vi "Get_PV-I.vi"(0 "CA Lab data":T2, 11 "Error in (no error)":errorcluster) -> (4 "PV Name (dup)":string, 6 "1rst Value (string)":string, 8 "1rst Value (number)":dbl, 10 "Value Array (number)":dbl[](array[numeric]), 13 "Status":bool, 14 "PV Info":T1[](array[typedef]), 15 "Error out":errorcluster)   [LabVIEW 2018]
doc: "This is a VI for reading values of EPICS variables.\n\nINPUT:\n <b>CA Lab data</b>\n Cluster with preinitialized data\n <b>Error in (no error)</b>\n\nOUTPUT:\n <b>PV Name (dup)</b>\n name array of EPICS variables\n <b>1st Value(string)</b>\n value of variable as String\n shows first item of value array\n <b>1st Value(number)</b>\n value of variable as Double\n shows first item of value array\n <b>Value Array(number)</b>\n all values of variable in Double array\n <b>Error out</b>\n <b>PV Info</b>\n cluster array of full answer\n value array(number)\n PV name\n elements\n size of value array\n value array(string)\n all values of variable in string array\n value array(number)\n elements\n size of value array\n status(string)\n status of EPICS PV as String\n status(number)\n status of EPICS PV as Long\n severity(string)\n severity of EPICS PV as String\n severity(number)\n severity of EPICS PV as Long\n time stamp(string)\n stamp of EPICS PV time as String\n time stamp(number)\n stamp of EPICS PV as Long\n field names\n field values\n string array of requsted EPICS field values\n error IO\n <b>Status</b>\n FALSE: request successful\n TRUE: warnings or errors"
uses:
  <userlib>/caLab/PV Info.ctl
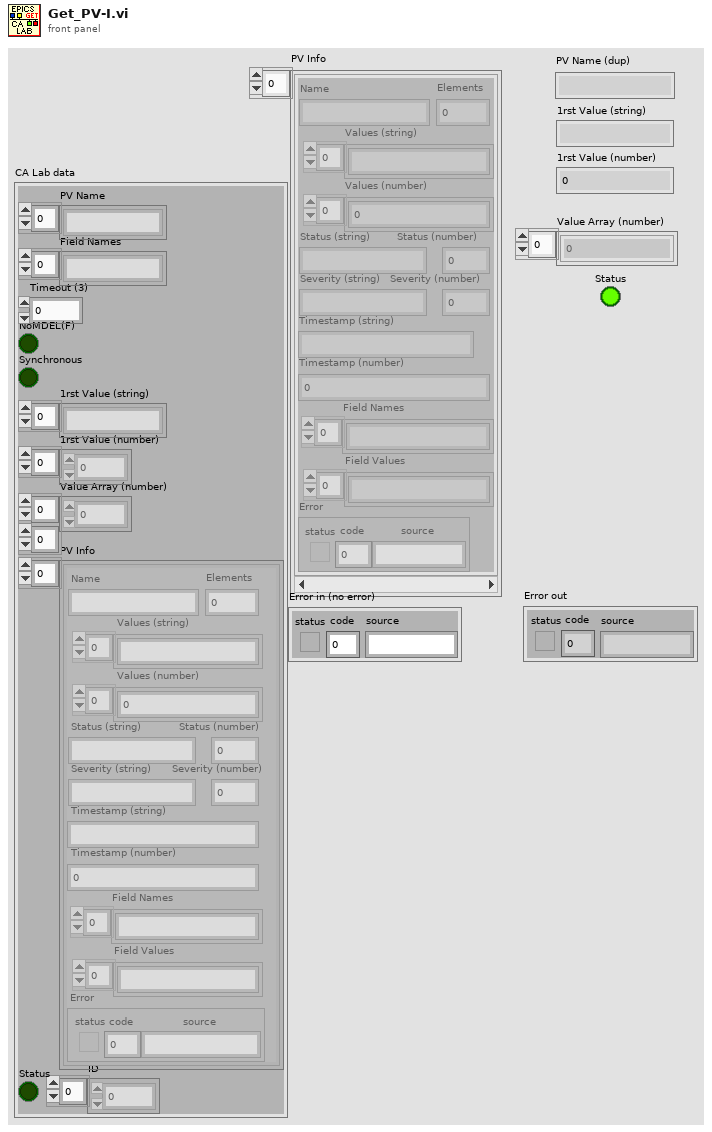
[diagram p1: front panel]
types:
  T1 = typedef "PV Info.ctl" = cluster{"Name":string, "Elements":i32, "Values (string)":string[], "Values (number)":dbl[], "Status (string)":string, "Status (number)":i16, "Severity (string)":string, "Severity (number)":i16, "Timestamp (string)":string, "Timestamp (number)":i32, "Field Names":string[], "Field Values":string[], "Error":errorcluster}
  T2 = cluster{"PV Name":string[], "Field Names":string[], "Timeout (3)":dbl, "NoMDEL(F)":bool, "Synchronous":bool, "1rst Value (string)":string[], "1rst Value (number)":dbl[], "Value Array (number)":dbl[][], "PV Info":T1[], "Status":bool, "ID":u64[]}
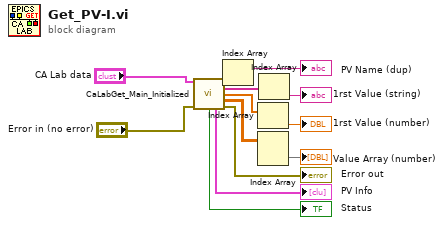
[diagram p0: block diagram]
diagram:
  n1 = call <userlib>:"CaLabGet_Main_Initialized.vi"("CA Lab data"="CA Lab data", "Error in (no error)"="Error in (no error)") -> ("PV Name (dup)"=w3:string[], "1rst Value (string)"=w9:string[], "1rst Value (number)"=w7:dbl[], "Value Array (number)"=w5:dbl[][], "Status"=→"Status":bool, "PV Info"=→"PV Info":T1[], "Error out"=→"Error out":errorcluster)  [unwired: 7 in]
  n2 = Index Array(array=w3) -> (element=→"PV Name (dup)":string)  [unwired: 1 in]
  n3 = Index Array(array=w7) -> (element=→"1rst Value (number)":dbl)  [unwired: 1 in]
  n4 = Index Array(array=w5) -> (element=→"Value Array (number)":dbl[])  [unwired: 2 in]
  n5 = Index Array(array=w9) -> (element=→"1rst Value (string)":string)  [unwired: 1 in]
